vi "Info.vi"() -> ()   [LabVIEW 2021]
panel:
  in  "Exit Button":bool caption="Cancel Button"
  in  "PTPS":bool
  in  "SWPS":bool
  # "Program służy do symulowania odpowiedzi czasowych oraz charakterystyk Silnika Wykonawczego Prądu Stałego oraz Prądnicy Tachometrycznej Prądu Stałego.\n\nProgram automatycznie wyświetla wykresy i aktualizuje je z każdą zmianą parametrów.\nSkala jest również automatycznie dopasowywana do minimalnych i maksymalnych wartości danych wejściowych. Istnieje możliwość wyłączenia tej opcji poprzez kliknięcię prawym przyciskiem myszy w wykres i odznaczenie odpowiedniego pola w wyświetlonym menu.\nParametry potrzebne do wygenerowania wykresów można wpisać za pomocą klawiatury bądź zmieniać przy użyciu strzałem widocznych na kontrolkach.\nAby zapisać wygenerowane dane, po naciśnięciu przycisku \"Zapisz\" należy w oknie systemowym wpisać nazwę pliku wraz z rozszerzeniem oraz wybrać lokalizację w której ma zostać utworzony plik. Program poprawnie obsługuje zapis do formatów .csv oraz .txt."
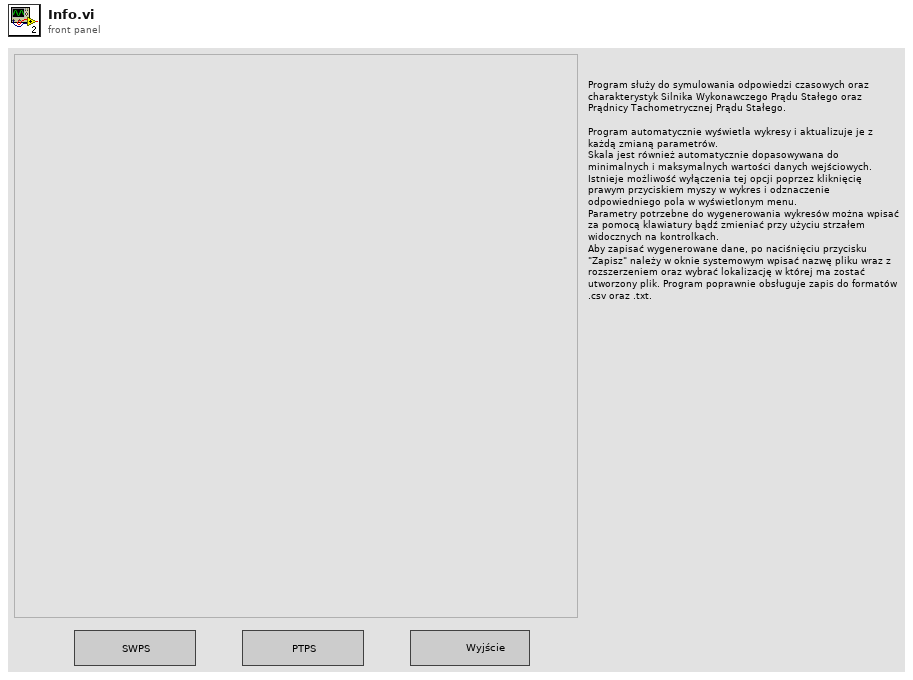
[diagram p1: front panel]
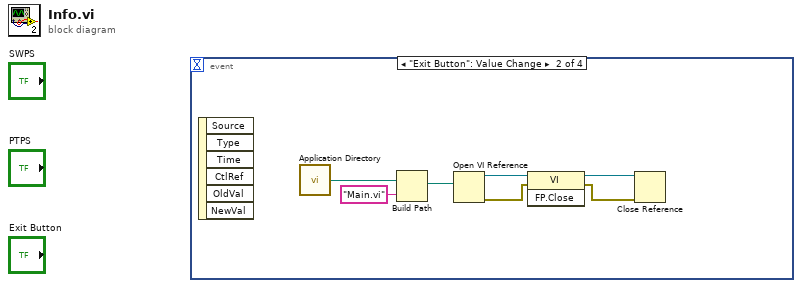
[diagram p0: block diagram]
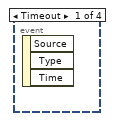
[diagram p2: hidden frame]
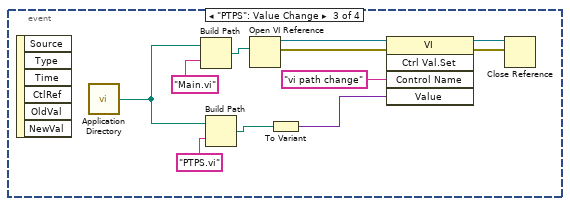
[diagram p3: hidden frame]
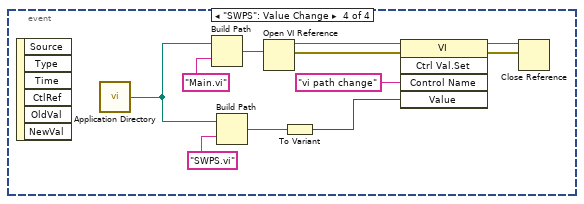
[diagram p4: hidden frame]
diagram:
  n1 = event shown="[1] \"Exit Button\": Value Change" {
    selector: _ -> [_ _ _ _]
    dyn-events: _ -> [_ _ _ _]
    timeout: _ -> [_ _ _ _]
    event Timeout {
      n2 = event-data() -> ()  [unwired: 1 in, 3 out]
    }
    event "Exit Button": Value Change {
      n3 = event-data() -> ()  [unwired: 1 in, 6 out]
      n4 = call <vilib>:"Application Directory.vi"() -> ("Application Directory"=w5:path)
      n5 = Build Path(base path=w5, name or relative path="Main.vi") -> (appended path=w6:path)
      n6 = Open VI Reference(vi path=w6) -> (vi reference=w4:refnum<vi>, error out=w2:errorcluster)  [unwired: 5 in]
      n7 = invoke class="VI" method="FP.Close"(reference=w4, error in=w2) -> (reference out=w3:refnum<vi>, error out=w1:errorcluster)  [unwired: 1 in, 1 out]
      n8 = Close Reference(reference=w3, error in (no error)=w1) -> ()  [unwired: 1 out]
    }
    event "PTPS": Value Change {
      n9 = event-data() -> ()  [unwired: 1 in, 6 out]
      n10 = call <vilib>:"Application Directory.vi"() -> ("Application Directory"=w10:path)
      n11 = Build Path(base path=w10, name or relative path="Main.vi") -> (appended path=w8:path)
      n12 = Build Path(base path=w10, name or relative path="PTPS.vi") -> (appended path=w9:path)
      n13 = Open VI Reference(vi path=w8) -> (vi reference=w16:refnum<vi>, error out=w15:errorcluster)  [unwired: 5 in]
      n14 = To Variant(anything=w9) -> (Variant=w13:variant)
      n15 = invoke class="VI" method="Ctrl Val.Set"(reference=w16, error in=w15, "Control Name"="vi path change", "Value"=w13) -> (reference out=w17:refnum<vi>, error out=w18:errorcluster)  [unwired: 1 in, 3 out]
      n16 = Close Reference(reference=w17, error in (no error)=w18) -> ()  [unwired: 1 out]
    }
    event "SWPS": Value Change {
      n17 = event-data() -> ()  [unwired: 1 in, 6 out]
      n18 = call <vilib>:"Application Directory.vi"() -> ("Application Directory"=w19:path)
      n19 = Build Path(base path=w19, name or relative path="Main.vi") -> (appended path=w22:path)
      n20 = Build Path(base path=w19, name or relative path="SWPS.vi") -> (appended path=w20:path)
      n21 = Open VI Reference(vi path=w22) -> (vi reference=w27:refnum<vi>, error out=w26:errorcluster)  [unwired: 5 in]
      n22 = To Variant(anything=w20) -> (Variant=w24:variant)
      n23 = invoke class="VI" method="Ctrl Val.Set"(reference=w27, error in=w26, "Control Name"="vi path change", "Value"=w24) -> (reference out=w28:refnum<vi>, error out=w29:errorcluster)  [unwired: 1 in, 3 out]
      n24 = Close Reference(reference=w28, error in (no error)=w29) -> ()  [unwired: 1 out]
    }
  }
